vi "Set Scaling Parameters.vi"   [LabVIEW 2020, in "SLSC.lvlib"]
doc: "Sets scaling parameters for a scale."
uses:
  <vilib>/SLSC/SLSC.lvlib
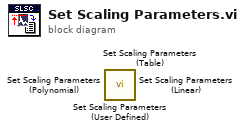
[diagram p0: block diagram]
diagram:
  n1 = call <vilib>:"Set Scaling Parameters (User Defined).vi"() -> ()  [unwired: 13 in, 3 out]
  n2 = call <vilib>:"Set Scaling Parameters (Table).vi"() -> ()  [unwired: 13 in, 3 out]
  n3 = call <vilib>:"Set Scaling Parameters (Polynomial).vi"() -> ()  [unwired: 13 in, 3 out]
  n4 = call <vilib>:"Set Scaling Parameters (Linear).vi"() -> ()  [unwired: 13 in, 3 out]
